vi "Initialize.vi"(8 "error in (no error)":errorcluster, 11 "DAQ Class in":refnum<class "DAQ Class.lvclass">) -> (0 "error out":errorcluster, 3 "DAQ Class out":refnum<class "DAQ Class.lvclass">)   [LabVIEW 2014, in "DAQ Class.lvclass"]
uses:
  DAQ Class.lvclass
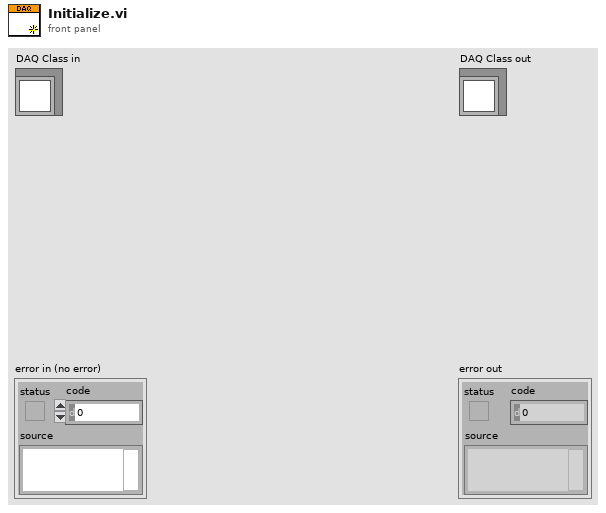
[diagram p1: front panel]
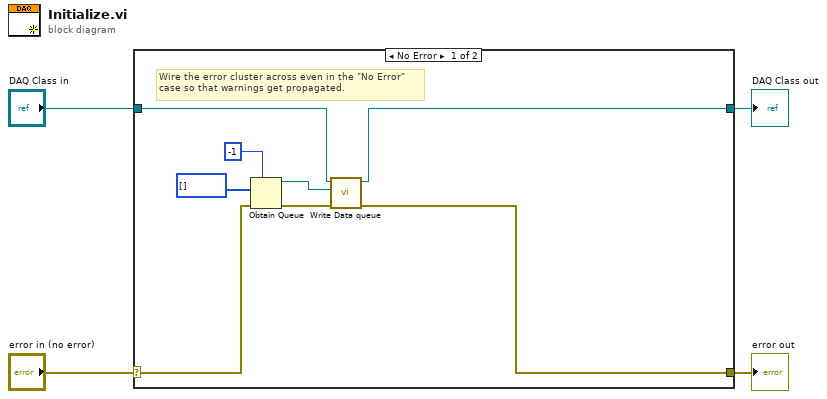
[diagram p0: block diagram]
diagram:
  n1 = case shown="No Error" "error in (no error)" {
    selector: "error in (no error)" -> [w9 w14]
    tunnel: [w6 w14] -> w3
    tunnel: [w5 w13] -> w1
    tunnel: "DAQ Class in" -> [w11 w13]
    frame No Error {
      # "Wire the error cluster across even in the \"No Error\"\ncase so that warnings get propagated."
      n2 = Obtain Queue(max queue size (-1, unlimited)=-1, element data type=u16[] [], error in (no error)=w9) -> (queue out=w12:refnum<queue>, error out=w7:errorcluster)  [unwired: 2 in, 1 out]
      n3 = call-dynamic "Write Data queue.vi"("error in (no error)"=w7, "Data queue"=w12, "DAQ Class in"=w11) -> ("error out"=w6:errorcluster, "DAQ Class out"=w5:refnum<class "DAQ Class.lvclass">)  [unwired: 7 in]
    }
    frame Error {
    }
  }
  "error out" <- w3
  "DAQ Class out" <- w1
